vi "Robot Main.vi"   [LabVIEW 2014]
doc: "This VI imlements the framework and scheduler for your robotics program. It should not be necessary to modify the framework. You are expected to add your code to the VIs called from Robot Main, the ones located in the Team Code within the project."
panel:
  # "2015 ÜberCode"
  # "Version 5.0.0  --  2015-03-08 -- Dartmouth"
  # "Solenoid"
  # "Controls"
  # "PWM"
  # "DIO"
  # "CAN"
  # "Relay"
  # "0: Front Right Wheel A\n 1: Front Right Wheel B\n 2: Front Left Wheel A\n 3: Front Left Wheel B\n 4: Center Wheel A\n 5: Center Wheel B\n 6: Back Left Wheel A\n 7: Back Left Wheel B\n 8: Back Right Wheel A\n 9: Back Right Wheel B\n MXP 0: Lift Belts A\n MXP 1: Lift Belts B\n MXP 2: Container Arm A\n MXP 3: Container Arm B\n MXP 4: Front Right Wheel A\n MXP 5: Front Right Wheel B"
  # "0: H-Drive Center Motor\n1: \n2: \n3: \n4: \n5:  \n6: \n7: \n8: \n9:"
  # "Joystick 1\nX Axis: Arcade/H-Drive Drive \nY Axis: Arcade/H-Drive Drive \nZ Axis:\nButton 1: Toggle Hold Position\nButton 2: To Driver Control\nButton 3: Home Gyroscope\nButton 4:\nButton 5: \nButton 6: \nButton 7: \nButton 8: \nButton 9: to H-Drive w/ Spin (when held)\nButton 10: \nButton 11: to H-Drive (when held)\nButton 12: to H-Drive w/ PID (when held)"
  # "Joystick 2\nX Axis: \nY Axis: Lift Up/Down\nZ Axis: \nButton 1: Toggle Lift Auto/DC \nButton 2: \nButton 3: \nButton 4: \nButton 5: \nButton 6: \nButton 7: \nButton 8: Lift Manual Override\nButton 9: Lift Index Up\nButton 10: \nButton 11: Lift Index Down\nButton 12:"
  # "Joystick 3\nX Axis: \nY Axis: Arm Up/Down \nZ Axis: \nButton 1: Toggle Arm Null/DC\nButton 2: \nButton 3: Retract Tote Pistons\nButton 4: \nButton 5: Extend Tote Pistons\nButton 6: \nButton 7: \nButton 8: Container Arm Manual\nButton 9: \nButton 10: \nButton 11: \nButton 12:"
  # "0:\n1:\n2:\n3:"
  # "0: \n1: \n2: \n3: \n4: \n5: \n6:\n7:"
  # "Power Distribution Panel\n - ID: 0\n\nPneumatics Control Module\n - ID: 0\n\nCAN Talon SRXs\n - Front Right ID: 1\n - Front Left ID: 2\n - Back Left ID: 3\n - Back Right ID: 4\n - Container Arm ID: 5\n - Lift Motor 1 ID: 6\n - Lift Motor 2 ID: 7"
  # "Analog"
  # "0: Gyroscope\n1: Gyroscope Temp.\n2:\n3:"
  # "PD Panel CAN Map"
  # "CH 8:"
  # "CH 9:"
  # "CH 10:"
  # "CH 11:"
  # "CH 12: Front Left Drive Motor"
  # "CH 13: Front Right Drive Motor"
  # "CH 14: Back Left Drive Motor"
  # "CH 15: Back Right Drive Motor"
  # "CH 7:"
  # "CH 6:"
  # "CH 5:"
  # "CH 4:"
  # "CH 0: Center Drive Motor"
  # "CH 1: Container Arm"
  # "CH 3: Lift Motor 2"
  # "CH 2: Lift Motor 1"
  # "POWER DISTRIBUTION PANEL"
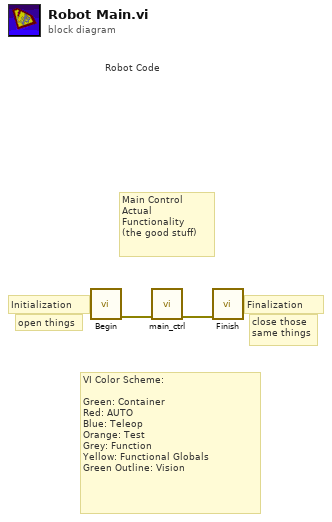
[diagram p0: block diagram]
diagram:
  # "Robot Code"
  # "close those\nsame things"
  # "open things"
  # "Finalization"
  # "Main Control\nActual Functionality\n(the good stuff)"
  # "Initialization"
  # "VI Color Scheme:\n\nGreen: Container\nRed: AUTO\nBlue: Teleop\nOrange: Test\nGrey: Function\nYellow: Functional Globals\nGreen Outline: Vision"
  n1 = call "Begin.vi"() -> ("Error Out"=w2:errorcluster)  [unwired: 7 in]
  n2 = call "main_ctrl.vi"("Error In"=w2) -> ("error out"=w1:errorcluster)  [unwired: 10 in]
  n3 = call "Finish.vi"("error in"=w1) -> ()  [unwired: 7 in]
